vi "RecursiveResultListTraversal.vi"(7 "report section in":refnum<k7>, 8 "error in (no error)":errorcluster, 9 "enable":bool, 10 "lookup string":string, 11 "property object in":refnum<k7>) -> (0 "error out":errorcluster, 3 "property object out":refnum<k7>, 5 "report section out":refnum<k7>)   [LabVIEW 2019]
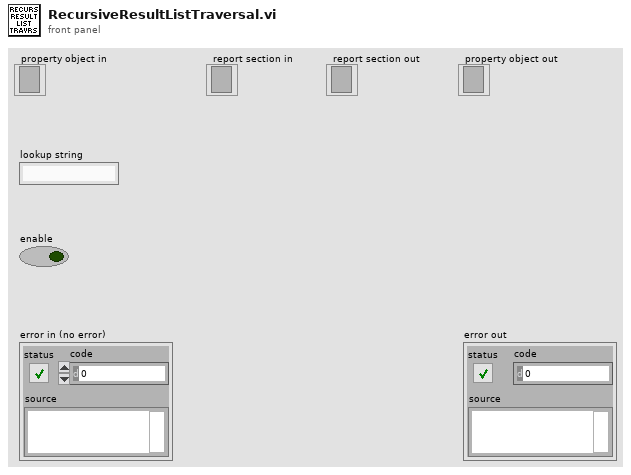
[diagram p1: front panel]
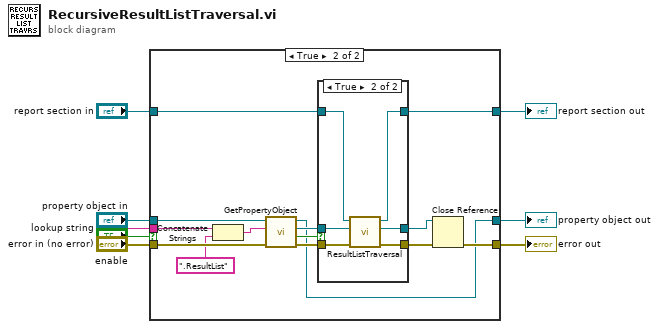
[diagram p0: block diagram]
diagram:
  n1 = case shown="True" "enable" {
    tunnel: "lookup string" -> [_ w24]
    tunnel: "property object in" -> [w9 w21]
    tunnel: "error in (no error)" -> [w10 w25]
    tunnel: "report section in" -> [w11 w17]
    tunnel: [w11 w16] -> w6
    tunnel: [w10 w13] -> w7
    tunnel: [w9 w12] -> w8
    frame False {
    }
    frame True {
      n2 = Concatenate Strings(w24, ".ResultList" ("string")) -> (w22:string)
      n3 = call "GetPropertyObject.vi"("error in (no error)"=w25, "lookup string"=w22, "property object in"=w21) -> ("error out"=w19:errorcluster, "exists"=w20:bool, "property object"=w18:refnum<k7>, "property object out"=w12:refnum<k7>)  [unwired: 5 in]
      n4 = case shown="True" w20 {
        tunnel: w19 -> [w26 w34]
        tunnel: w18 -> [w27 w33]
        tunnel: w17 -> [w28 w32]
        tunnel: [w28 w31] -> w16
        tunnel: [w27 w30] -> w15
        tunnel: [w26 w29] -> w14
        frame False {
        }
        frame True {
          n5 = call "ResultListTraversal.vi"("error in (no error)"=w34, "result list in"=w33, "report section in"=w32) -> ("error out"=w29:errorcluster, "result list out"=w30:refnum<k7>, "report section out"=w31:refnum<k7>)  [unwired: 6 in]
        }
      }
      n6 = Close Reference(reference=w15, error in (no error)=w14) -> (error out=w13:errorcluster)
    }
  }
  "property object out" <- w8
  "error out" <- w7
  "report section out" <- w6
